vi "Attitude_Display_Pascal_Kolleg.vi"() -> (2 "TdxCopter":refnum<vi>)   [LabVIEW 2013]
uses:
  <vilib>/Utility/miscctls.llb/LV3DPointTypeDef.ctl
  <vilib>/picture/3D Picture Control/Object/Create Object (name).vi
  <vilib>/picture/3D Picture Control/NI_3D Picture Control.lvlib
panel:
  out "3D Picture":refnum<vi>(3d-picture)
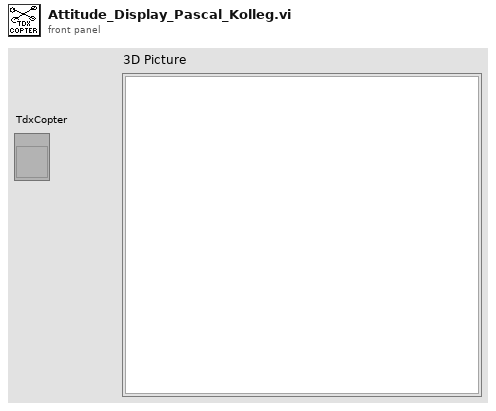
[diagram p1: front panel]
types:
  T1 = typedef "LV3DPointTypeDef.ctl" = cluster{"X":sgl, "Y":sgl, "Z":sgl}
  T2 = cluster{"Red":sgl, "Green":sgl, "Blue":sgl, "Alpha":sgl}
  T3 = cluster{"Red":sgl, "Green":sgl, "Blue":sgl, "Alpha":sgl}[]
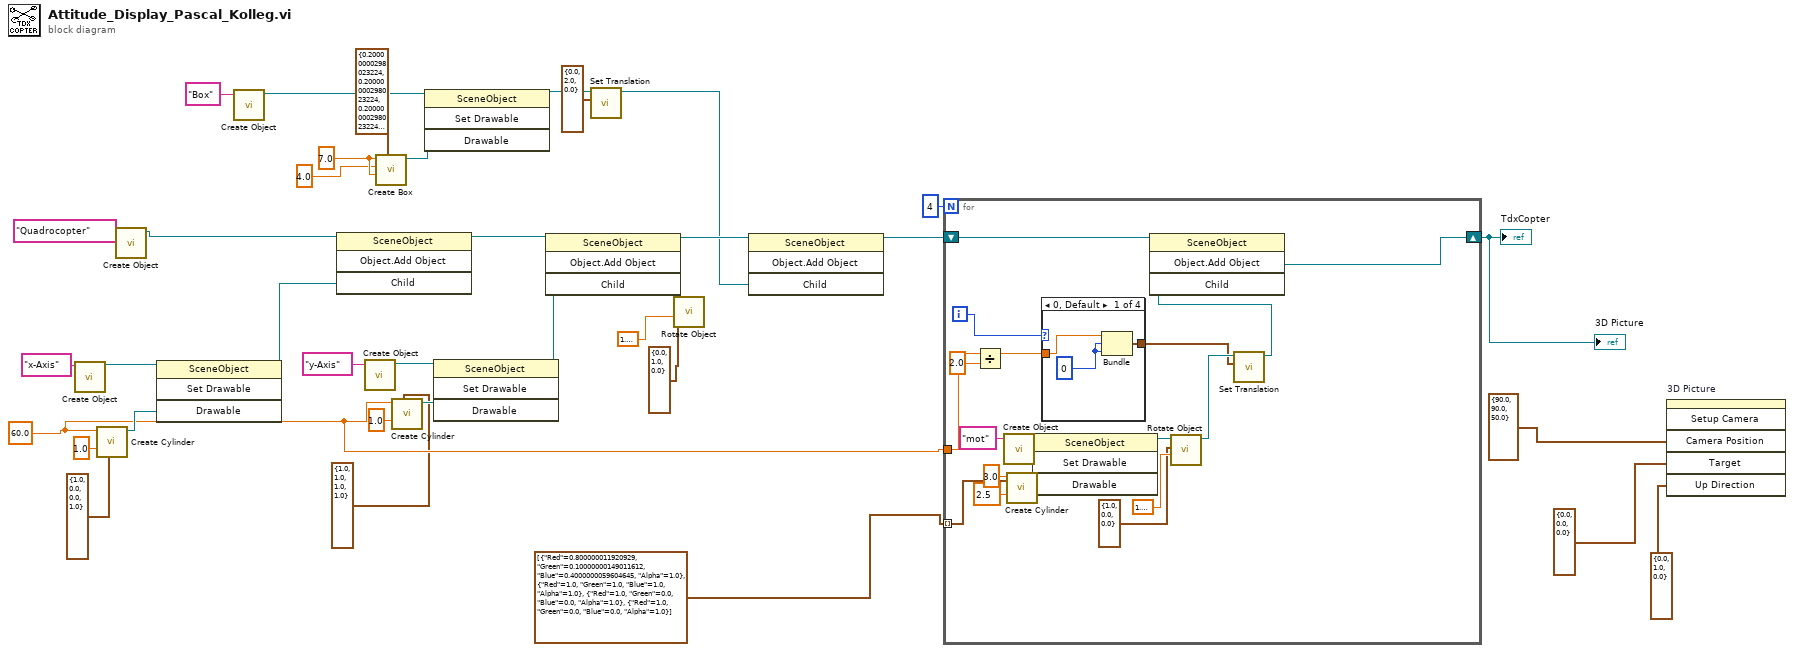
[diagram p0: block diagram]
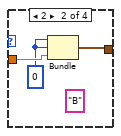
[diagram p2: hidden frame]
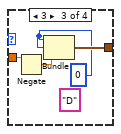
[diagram p3: hidden frame]
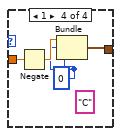
[diagram p4: hidden frame]
diagram:
  w6 = sgl 7.0 ("Length X")
  w19 = sgl 60.0 ("Height")
  n1 = call-poly <vilib>:"Create Object.vi"("Name"="x-Axis") -> ("Scene:New Object"=w25:refnum<vi>)  [unwired: 9 in, 1 out]
  n2 = call <vilib>:"Create Cylinder.vi"("Color"=T2 {"Red"=1.0, "Green"=0.0, "Blue"=0.0, "Alpha"=1.0}, "Radius"=sgl 1.0, "Height"=w19) -> ("New Cylinder Refnum"=w26:refnum<vi>)  [unwired: 7 in, 1 out]
  n3 = call-poly <vilib>:"Create Object.vi"("Name"="Quadrocopter") -> ("Scene:New Object"=w22:refnum<vi>)  [unwired: 9 in, 1 out]
  n4 = invoke class="SceneObject" method="Set Drawable"(reference=w25, "Drawable"=w26) -> (reference out=w23:refnum<vi>)  [unwired: 2 in, 3 out]
  n5 = call-poly <vilib>:"Create Object.vi"("Name"="Box") -> ("Scene:New Object"=w13:refnum<vi>)  [unwired: 9 in, 1 out]
  n6 = invoke class="SceneObject" method="Object.Add Object"(reference=w22, "Child"=w23) -> (reference out=w24:refnum<vi>)  [unwired: 2 in, 3 out]
  n7 = call-poly <vilib>:"Create Object.vi"("Name"="y-Axis") -> ("Scene:New Object"=w31:refnum<vi>)  [unwired: 9 in, 1 out]
  n8 = call <vilib>:"Create Box.vi"("Color"=T2 {"Red"=0.2, "Green"=0.2, "Blue"=0.2, "Alpha"=1.0}, "Length Z"=w6, "Length Y"=sgl 4.0 ("Length Z"), "Length X"=w6) -> ("New Box Refnum"=w10:refnum<vi>)  [unwired: 6 in, 1 out]
  n9 = call <vilib>:"Create Cylinder.vi"("Color"=T2 {"Red"=1.0, "Green"=1.0, "Blue"=1.0, "Alpha"=1.0}, "Radius"=sgl 1.0, "Height"=w19) -> ("New Cylinder Refnum"=w32:refnum<vi>)  [unwired: 7 in, 1 out]
  n10 = invoke class="SceneObject" method="Set Drawable"(reference=w13, "Drawable"=w10) -> (reference out=w9:refnum<vi>)  [unwired: 2 in, 3 out]
  n11 = invoke class="SceneObject" method="Set Drawable"(reference=w31, "Drawable"=w32) -> (reference out=w33:refnum<vi>)  [unwired: 2 in, 3 out]
  n12 = invoke class="SceneObject" method="Object.Add Object"(reference=w24, "Child"=w33) -> (reference out=w12:refnum<vi>, "Child"=w34:refnum<vi>)  [unwired: 2 in, 2 out]
  n13 = call <vilib>:"Set Translation.vi"("Translation"=cluster{"X":sgl, "Y":sgl, "Z":sgl} {"X"=0.0, "Y"=2.0, "Z"=0.0}, "Scene Object"=w9) -> ("Translated Object"=w8:refnum<vi>)  [unwired: 8 in, 1 out]
  n14 = call <vilib>:"Rotate Object.vi"("Angle"=1.5707963267948966, "Axis"=cluster{"X":sgl, "Y":sgl, "Z":sgl} {"X"=0.0, "Y"=1.0, "Z"=0.0}, "Scene.Object In"=w34) -> ()  [unwired: 1 in, 8 out]
  n15 = invoke class="SceneObject" method="Object.Add Object"(reference=w12, "Child"=w8) -> (reference out=w11:refnum<vi>)  [unwired: 2 in, 3 out]
  n16 = for {
    N: 4 -> [_]
    shift-right: [w37] -> w4
    shift-left: w11 -> [w54]
    tunnel: w19 -> [w46]
    tunnel: T3 [{"Red"=0.8, "Green"=0.1, "Blue"=0.4, "Alpha"=1.0}, {"Red"=1.0, "Green"=1.0, "Blue"=1.0, "Alpha"=1.0}, {"Red"=1.0, "Green"=0.0, "Blue"=0.0, "Alpha"=1.0}, {"Red"=1.0, "Green"=0.0, "Blue"=0.0, "Alpha"=1.0}] -> [w39] mode=indexing
    i -> [w45]
    n17 = Divide(x=w46, y=sgl 2.0) -> (x/y=w41:sgl)
    n18 = call-poly <vilib>:"Create Object.vi"("Name"="mot") -> ("Scene:New Object"=w50:refnum<vi>)  [unwired: 9 in, 1 out]
    n19 = call <vilib>:"Create Cylinder.vi"("Color"=w39, "Radius"=sgl 2.5, "Height"=sgl 3.0) -> ("New Cylinder Refnum"=w49:refnum<vi>)  [unwired: 7 in, 1 out]
    n20 = invoke class="SceneObject" method="Set Drawable"(reference=w50, "Drawable"=w49) -> (reference out=w48:refnum<vi>)  [unwired: 2 in, 3 out]
    n21 = case shown="0, Default" w45 {
      tunnel: w41 -> [w56 w59 w63 w67]
      tunnel: [w57 w60 w64 w68] -> w38
      frame 0, Default {
        w55 = 0
        n22 = Bundle(w56, w55, w55) -> (w57:cluster{sgl, i32, i32})  [unwired: 1 in]
      }
      frame 2 {
        (unwired) "B" ("Name")
        w58 = 0
        n23 = Bundle(w58, w58, w59) -> (w60:cluster{i32, i32, sgl})  [unwired: 1 in]
      }
      frame 3 {
        (unwired) "D" ("Name")
        w61 = 0
        n24 = Negate(x=w63) -> (-x=w62:sgl)
        n25 = Bundle(w61, w61, w62) -> (w64:cluster{i32, i32, sgl})  [unwired: 1 in]
      }
      frame 1 {
        (unwired) "C" ("Name")
        w65 = 0
        n26 = Negate(x=w67) -> (-x=w66:sgl)
        n27 = Bundle(w66, w65, w65) -> (w68:cluster{sgl, i32, i32})  [unwired: 1 in]
      }
    }
    n28 = call <vilib>:"Rotate Object.vi"("Angle"=1.5707963267948966, "Axis"=cluster{"X":sgl, "Y":sgl, "Z":sgl} {"X"=1.0, "Y"=0.0, "Z"=0.0}, "Scene.Object In"=w48) -> ("Scene.Object Out"=w47:refnum<vi>)  [unwired: 1 in, 7 out]
    n29 = call <vilib>:"Set Translation.vi"("Translation"=w38, "Scene Object"=w47) -> ("Translated Object"=w44:refnum<vi>)  [unwired: 8 in, 1 out]
    n30 = invoke class="SceneObject" method="Object.Add Object"(reference=w54, "Child"=w44) -> (reference out=w37:refnum<vi>)  [unwired: 2 in, 3 out]
  }
  "TdxCopter" <- w4
  "3D Picture" <- w4
  n31 = invoke on="3D Picture" class="SceneGraphDisp (strict)" method="Setup Camera"("Camera Position"=T1 {"X"=90.0, "Y"=90.0, "Z"=50.0}, "Target"=T1 {"X"=0.0, "Y"=0.0, "Z"=0.0}, "Up Direction"=T1 {"X"=0.0, "Y"=1.0, "Z"=0.0}) -> ()  [unwired: 3 in, 6 out]
